vi "PicohrdlGetValues.vi"(5 "noOfValues":i32=20, 7 "Channel Enable Array":u8[](array[numeric]), 8 "error in (no error)":errorcluster, 9 "noOfChannels":i16=1, 10 "Buffer size":i32=1000, 11 "Handle in":i16) -> (0 "error out":errorcluster, 1 "Overflow":i16 format="%020b", 2 "temp_buffer":i32[](array[numeric]), 3 "Handle out":i16)   [LabVIEW 2010]
doc: "Calls HRDLGetValues() to retieve data from unit."
uses:
  PicoHRDL.dll
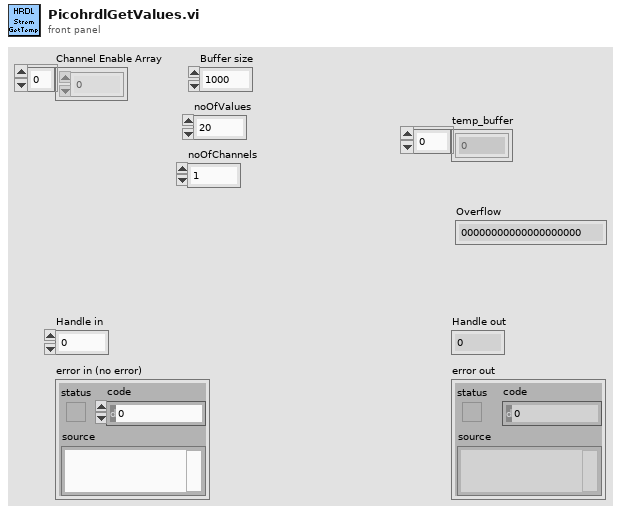
[diagram p1: front panel]
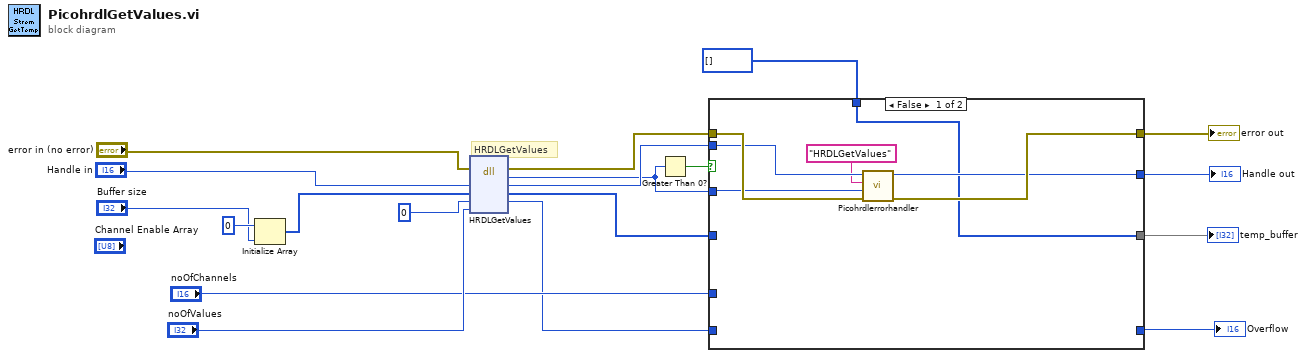
[diagram p0: block diagram]
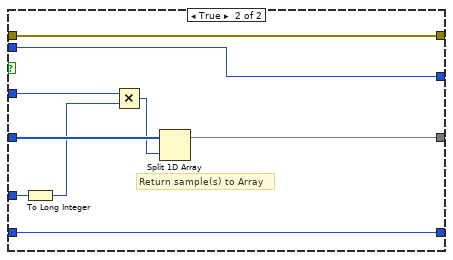
[diagram p2: hidden frame]
diagram:
  # "HRDLGetValues"
  n1 = Initialize Array(0 ("element"), "Buffer size") -> (w11:i32[])
  n2 = dll-call lib="PicoHRDL.dll" fn="HRDLGetValues"(error in="error in (no error)", "handle"="Handle in", "values"=w11, "overflow"=i16 0, "noOfValues"="noOfValues") -> (error out=w7:errorcluster, "noValuesPerChan"=w4:i32, "handle"=w6:i16, "values"=w8:i32[], "overflow"=w1:i16)  [unwired: 3 in, 1 out]
  n3 = Greater Than 0?(x=w4) -> (x > 0?=w5:bool)
  n4 = case shown="False" w5 {
    tunnel: w6 -> [w25 w35]
    tunnel: [w23 w35] -> w16
    tunnel: [w21 w27] -> w17
    tunnel: [w24 w34] -> w19
    tunnel: w7 -> [w26 w34]
    tunnel: w1 -> [_ w33]
    tunnel: [_ w33] -> w14
    tunnel: w4 -> [w20 w32]
    tunnel: w8 -> [_ w31]
    tunnel: "noOfChannels" -> [_ w28]
    tunnel: i32[] [] ("array") -> [w21 _]
    frame False {
      n5 = call "Picohrdlerrorhandler.vi"("Handle in"=w25, "API function"="HRDLGetValues", "Return"=w20, "error in (no error)"=w26) -> ("Handle out"=w23:i16, "error out"=w24:errorcluster)  [unwired: 5 in]
    }
    frame True {
      # "Return sample(s) to Array"
      n6 = To Long Integer(number=w28) -> (32bit integer=w29:i32)
      n7 = Multiply(x=w32, y=w29) -> (x*y=w30:i32)
      n8 = Split 1D Array(array=w31, index=w30) -> (first subarray=w27:i32[])  [unwired: 1 out]
    }
  }
  "error out" <- w19
  "temp_buffer" <- w17
  "Handle out" <- w16
  "Overflow" <- w14
